vi "Handle Error.vi"(8 "error in (no error)":errorcluster, 11 "UI Root in":refnum<class "UI Root.lvclass">) -> (0 "error out":errorcluster, 2 "stop actor?":bool=TRUE, 3 "UI Root out":refnum<class "UI Root.lvclass">)   [LabVIEW 2020, in "UI Root.lvlib" / "UI Root.lvclass"]
doc: "<p>(<strong>Filename</strong>: <span class=\"dnl\">Actor Framework.lvlib:Actor.lvclass:Handle Error.vi</span>)</p>\n<p>Defines how the actor handles an error that occurred while processing a message. By default, this method does nothing except stop the actor.</p>"
uses:
  UI Root.lvclass
  <vilib>/MGI/Panel Manager/Panel Actor/Panel Actor/Panel Actor.lvclass
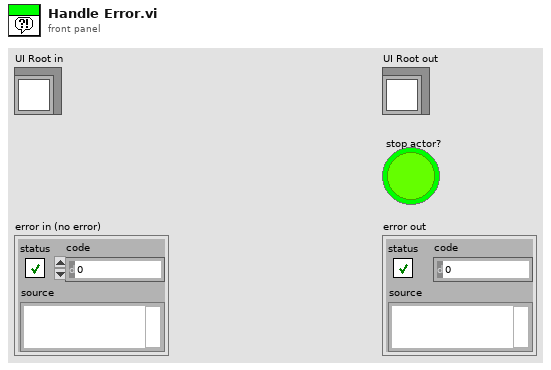
[diagram p1: front panel]
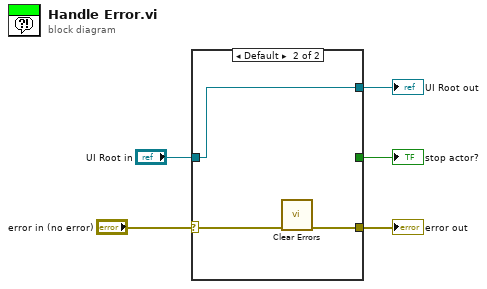
[diagram p0: block diagram]
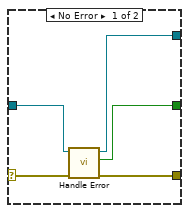
[diagram p2: hidden frame]
diagram:
  n1 = case shown="Default" "error in (no error)" {
    selector: "error in (no error)" -> [w7 w12]
    tunnel: [w10 w11] -> w5
    tunnel: [w9 _] -> w4
    tunnel: [w8 w13] -> w3
    tunnel: "UI Root in" -> [w6 w13]
    frame No Error {
      n2 = call-parent "Handle Error.vi"("error in (no error)"=w7, "Actor in"=w6) -> ("error out"=w10:errorcluster, "stop actor?"=w9:bool, "Actor out"=w8:refnum<class "UI Root.lvclass">)  [unwired: 7 in]
    }
    frame Default {
      n3 = call <vilib>:"Clear Errors.vi"("error in (no error)"=w12) -> ("error out"=w11:errorcluster)  [unwired: 5 in, 1 out]
    }
  }
  "UI Root out" <- w3
  "error out" <- w5
  "stop actor?" <- w4
